vi "WriteCalibrationVolumesToTable.vi"(11 "Table in":refnum<vi>) -> ()   [LabVIEW 2012]
uses:
  GlobalVariables/CalibrationVolumes.vi
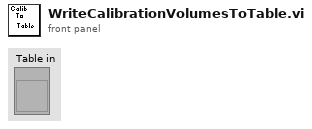
[diagram p1: front panel]
types:
  T1 = cluster{"CalibrationVolumes":dbl[], "SetName":string}[]
  T2 = cluster{"CalibrationVolumes":dbl[], "SetName":string}
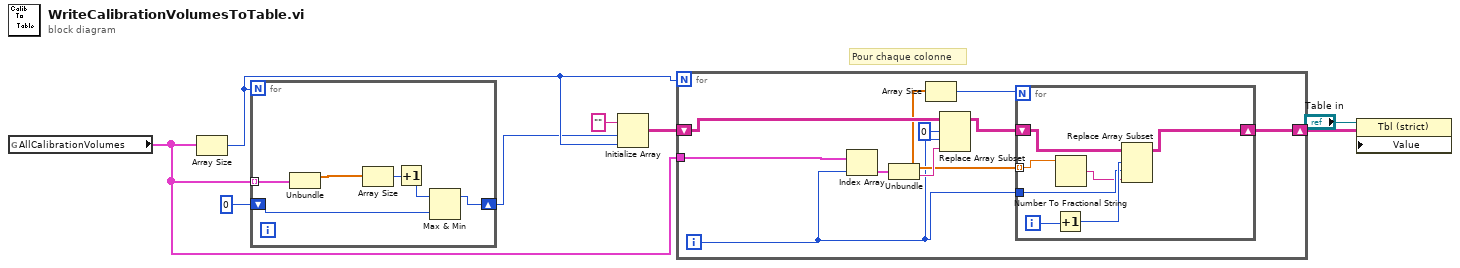
[diagram p0: block diagram]
diagram:
  # "Pour chaque colonne"
  n1 = global read "CalibrationVolumes.vi" "AllCalibrationVolumes"() -> (w8:T1)
  n2 = Array Size(array=w8) -> (size(s)=w5:i32)
  n3 = for {
    N: w5 -> [_]
    tunnel: w8 -> [w14] mode=indexing
    shift-right: [w11] -> w4
    shift-left: 0 -> [w12]
    n4 = Unbundle(w14) -> ("CalibrationVolumes"=w13:dbl[])  [unwired: 1 out]
    n5 = Array Size(array=w13) -> (size(s)=w10:i32)
    n6 = Increment(x=w10) -> (x+1=w9:i32)
    n7 = Max & Min(x=w9, y=w12) -> (max(x,y)=w11:i32)  [unwired: 1 out]
  }
  n8 = Initialize Array("", w4, w5) -> (w6:string[][])
  n9 = for {
    N: w5 -> [_]
    shift-right: [w19] -> w7
    shift-left: w6 -> [w23]
    tunnel: w8 -> [w15]
    i -> [w16]
    n10 = Index Array(array=w15, index=w16) -> (element=w24:T2)
    n11 = Unbundle(w24) -> ("CalibrationVolumes"=w17:dbl[], "SetName"=w21:string)
    n12 = Array Size(array=w17) -> (size(s)=w18:i32)
    n13 = Replace Array Subset(array=w23, new element=w21, index (row)=0, index (col)=w16) -> (w20:string[][])
    n14 = for {
      N: w18 -> [_]
      shift-right: [w30] -> w19
      shift-left: w20 -> [w31]
      tunnel: w17 -> [w26] mode=indexing
      tunnel: w16 -> [w27]
      i -> [w29]
      n15 = Increment(x=w29) -> (x+1=w28:i32)
      n16 = Number To Fractional String(number=w26) -> (F-format string=w25:string)  [unwired: 3 in]
      n17 = Replace Array Subset(array=w31, new element=w25, index (row)=w28, index (col)=w27) -> (w30:string[][])
    }
  }
  n18 = property class="Tbl (strict)"(reference="Table in", "Value"=w7) -> ()  [unwired: 1 in, 2 out]
